vi "HoloPy_template.vi"() -> ()   [LabVIEW 2023, in "holoPyTracks.lvlib"]
uses:
  holoPyTracks.lvlib
  subVis/HologramInfo.ctl
  subVis/analyse_parameters.ctl
panel:
  in  "analyse parameters":T1={"propagation"={"distance ini"=0.0, "number of planes"=0, "step"=0.0}, "Focus"={"Type"=enum."SUM_OF_INTENSITY", "Sum size"=1}, "Binarisation"={"Threshold ( N x Standard deviation)"=1.0, "Computed on"=enum."1st hologram"}, "CCL"={"Connectivity"=enum."6", "min voxel"=1.0, "max voxel"=1.0}, "Fourier BP filter (pix)"={"High pass (0=none)"=0.0, "Low Pass (0=none)"=0.0}} {"Fourier BP filter (pix)"."Low Pass (0=none)" format="%#_6e"; "CCL"."max voxel" min=1.0 max=100.0; "CCL"."min voxel" min=1.0 max=100.0; "Binarisation"."Threshold ( N x Standard deviation)" min=1.0 max=100.0; "Focus"."Sum size" min=1 max=100; "propagation"."step" format="%#_6e"; "propagation"."distance ini" format="%#_6e"}
  in  "HOLO INFO":T2 {"Holo size X" format="%#_6e"; "wavelength" format="%#_6e"}
  out "return value":string
  in  "Refnum in":refnum<k35>
  out "Refnum out":refnum<k35>
  in  "error in (no error)":errorcluster
  out "error out":errorcluster
  in  "Application Directory":path
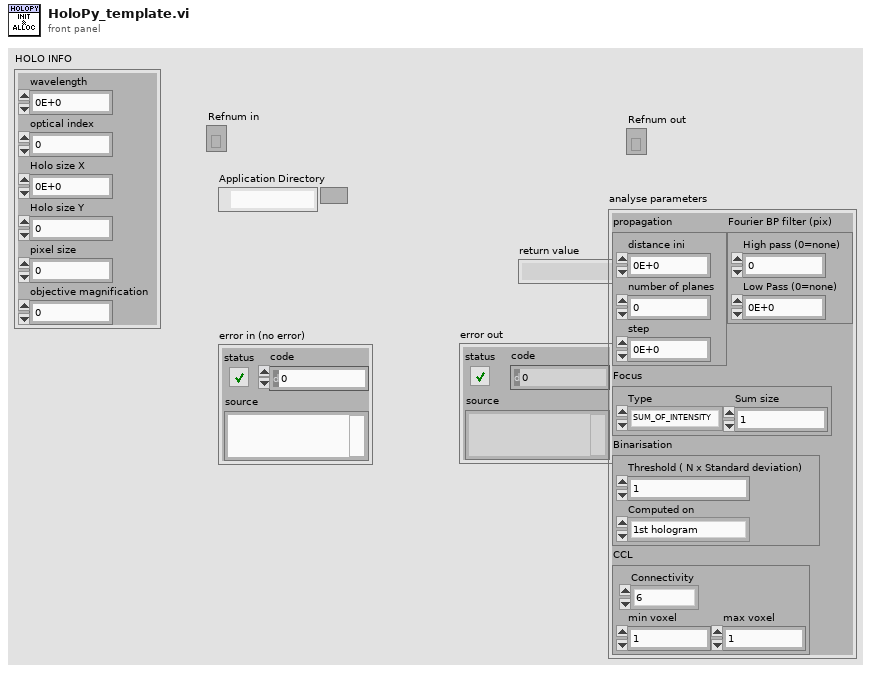
[diagram p1: front panel]
types:
  T1 = typedef "holoPyTracks.lvlib/analyse_parameters.ctl" = cluster{"propagation":cluster{"distance ini":dbl, "number of planes":i32, "step":dbl}, "Focus":cluster{"Type":enum16{"SUM_OF_INTENSITY", "SUM_OF_LAPLACIAN", "SUM_OF_VARIANCE", "TENENGRAD"}, "Sum size":i32}, "Binarisation":cluster{"Threshold ( N x Standard deviation)":dbl, "Computed on":enum16{"1st hologram", "each hologram"}}, "CCL":cluster{"Connectivity":enum16{"6", "18", "26"}, "min voxel":dbl, "max voxel":dbl}, "Fourier BP filter (pix)":cluster{"High pass (0=none)":dbl, "Low Pass (0=none)":dbl}}
  T2 = typedef "holoPyTracks.lvlib/HologramInfo.ctl" = cluster{"wavelength":sgl, "optical index":sgl, "Holo size X":i32, "Holo size Y":i32, "pixel size":sgl, "objective magnification":sgl}
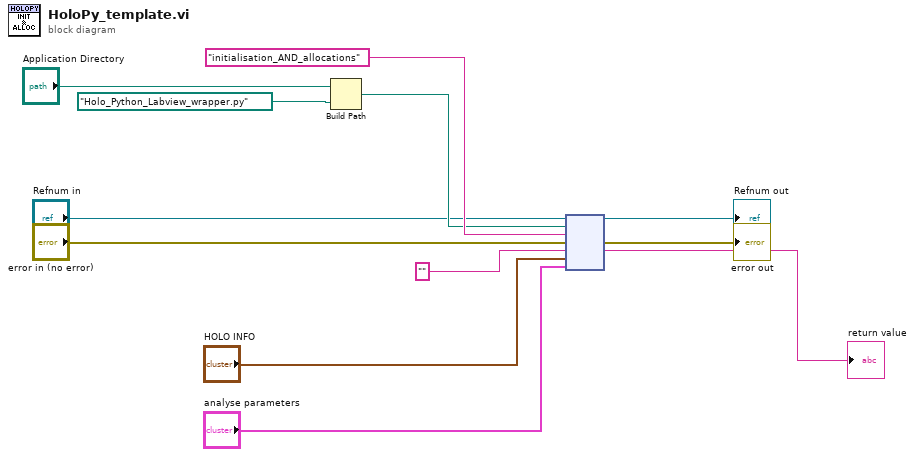
[diagram p0: block diagram]
diagram:
  n1 = Build Path(base path="Application Directory", name or relative path=path "Holo_Python_Labview_wrapper.py") -> (appended path=w11:path)
  n2 = node("Refnum in", w11, "initialisation_AND_allocations" ("function name"), "error in (no error)", "", "HOLO INFO", "analyse parameters") -> (→"Refnum out":refnum<k35>, →"error out":errorcluster, →"return value":string)  [unwired: 2 in, 2 out]
